vi "FilterRowData.vi"(4 "Row Filter":T1, 5 "error in (no error)":errorcluster, 7 "Ignore?":bool, 8 "Row XML Node":refnum<k20>) -> (0 "error out":errorcluster, 1 "Number Out":i32, 2 "Row Data":string[](array[string]), 3 "XML Node Out":refnum<k20>)   [LabVIEW 2013]
uses:
  RowDataFilter.ctl
  XML.lvlib
  <resource>/objmgr/DOMUserDefRef.rc
panel:
  # "Input"
  # "Output"
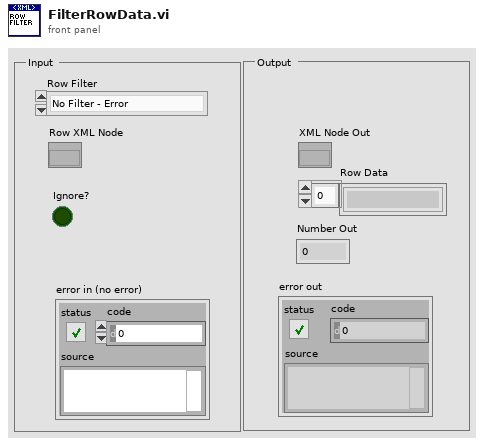
[diagram p1: front panel]
types:
  T1 = typedef "RowDataFilter.ctl" = enum16{"No Filter - Error", "Row Values", "Row Data", "#Rows Repeated", "#Columns Repeated"}
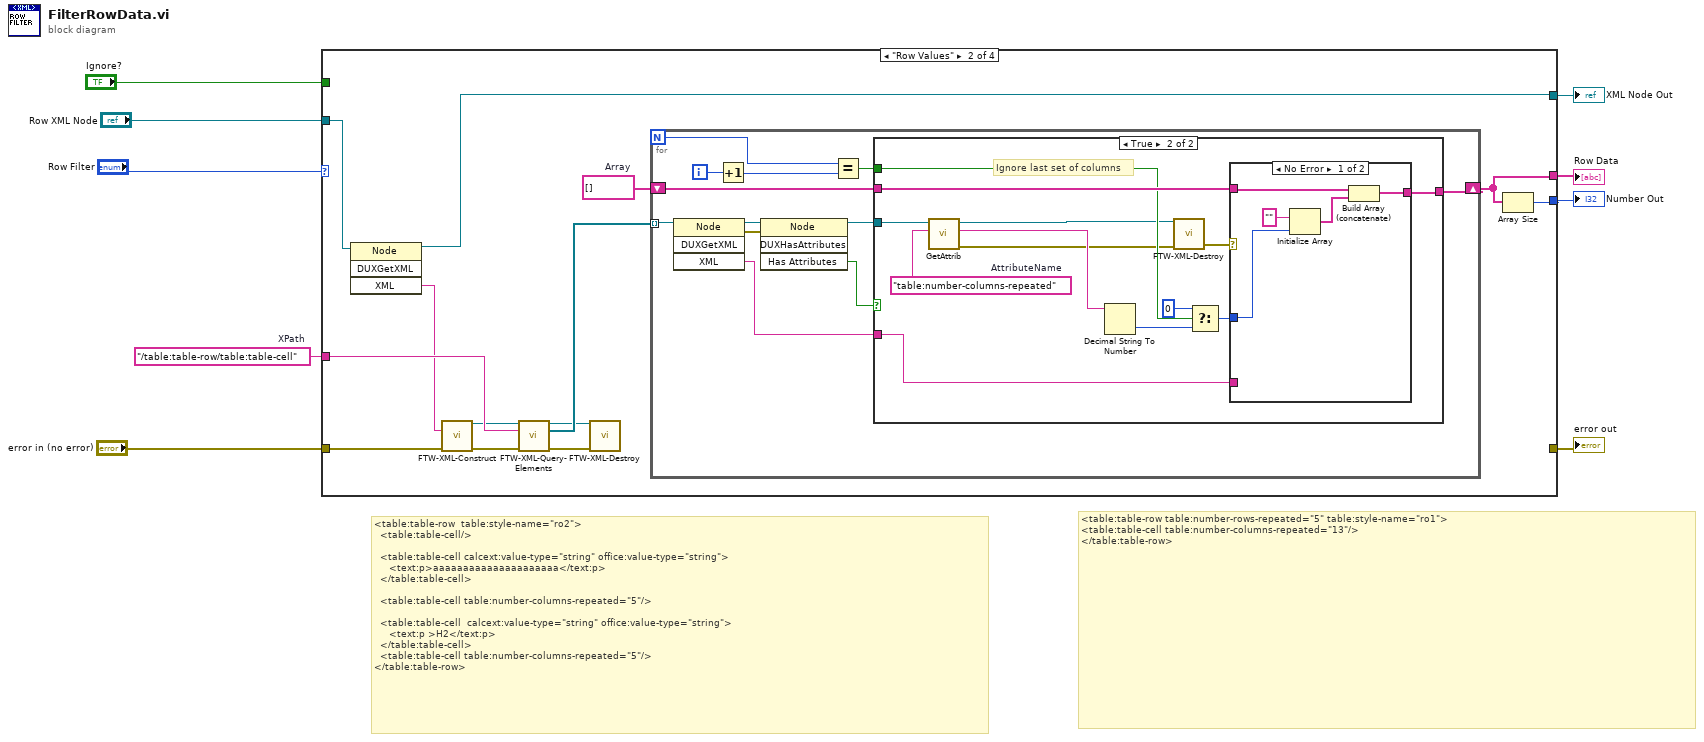
[diagram p0: block diagram]
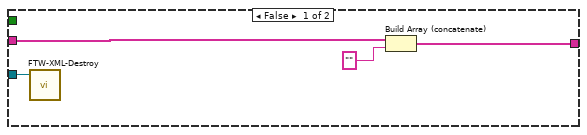
[diagram p3: hidden frame]
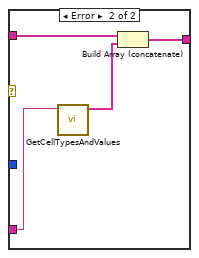
[diagram p4: hidden frame]
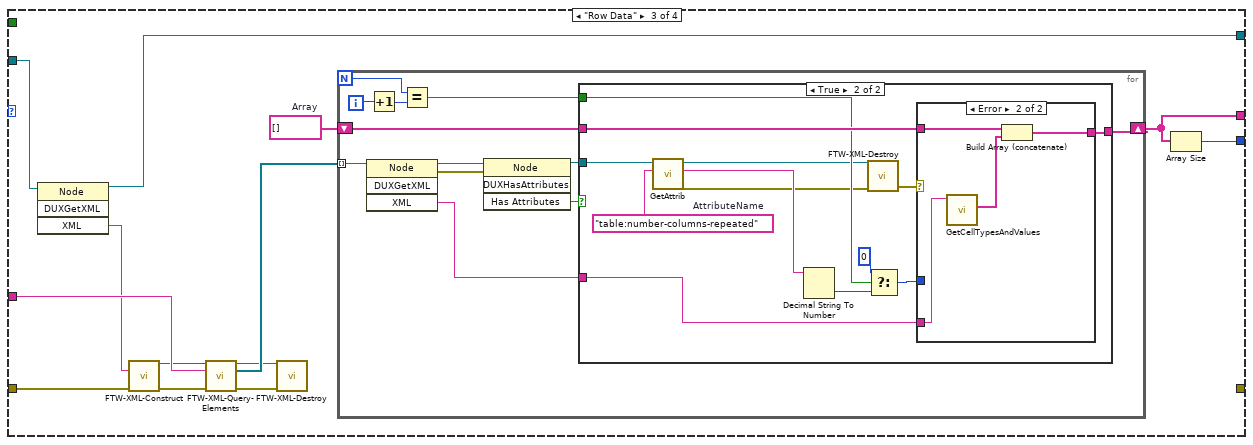
[diagram p5: hidden frame]
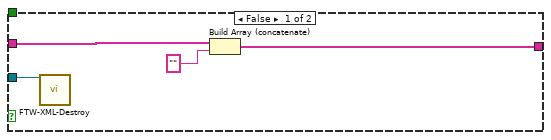
[diagram p6: hidden frame]
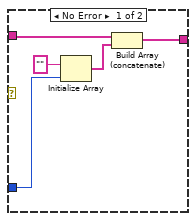
[diagram p7: hidden frame]
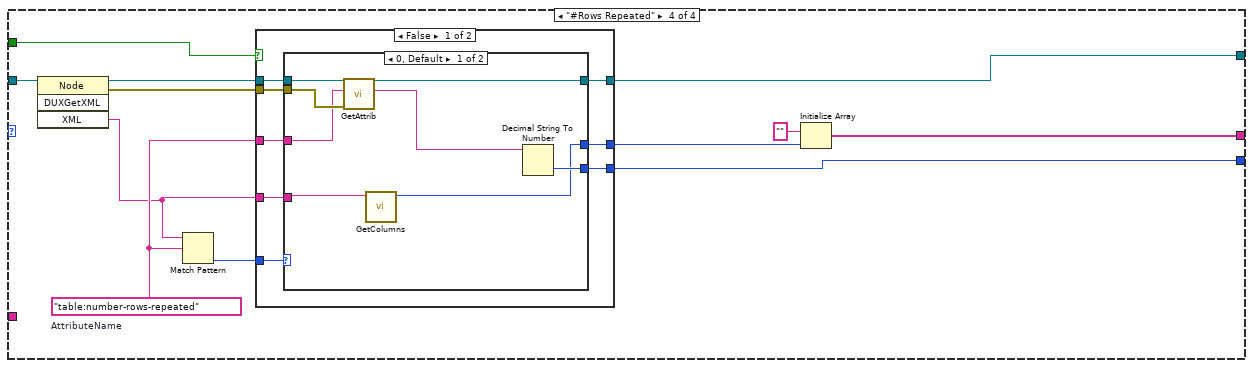
[diagram p8: hidden frame]
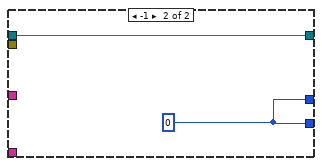
[diagram p9: hidden frame]
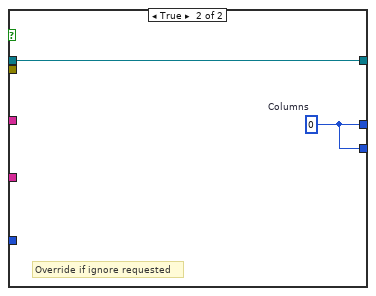
[diagram p10: hidden frame]
diagram:
  w1 = "/table:table-row/table:table-cell"  # XPath
  # "<table:table-row table:number-rows-repeated=\"5\" table:style-name=\"ro1\">\n<table:table-cell table:number-columns-repeated=\"13\"/>\n</table:table-row>"
  # "<table:table-row  table:style-name=\"ro2\">\n  <table:table-cell/>\n  \n  <table:table-cell calcext:value-type=\"string\" office:value-type=\"string\">           \n     <text:p>aaaaaaaaaaaaaaaaaaaaa</text:p>\n  </table:table-cell>\n  \n  <table:table-cell table:number-columns-repeated=\"5\"/>\n  \n  <table:table-cell  calcext:value-type=\"string\" office:value-type=\"string\">\n     <text:p >H2</text:p>\n  </table:table-cell>\n  <table:table-cell table:number-columns-repeated=\"5\"/>\n</table:table-row>"
  n1 = case shown="\"Row Values\"" "Row Filter" {
    tunnel: "error in (no error)" -> [w10 w17 w68 _]
    tunnel: "Row XML Node" -> [w11 w16 w67 w125]
    tunnel: [w11 w14 w65 w120] -> w6
    tunnel: [w10 _ _ _] -> w5
    tunnel: w1 -> [_ w24 w75 _]
    tunnel: [_ w21 w72 w122] -> w4
    tunnel: [_ w20 w71 w121] -> w3
    tunnel: "Ignore?" -> [_ _ _ w114]
    frame "No Filter - Error", Default {
    }
    frame "Row Values" {
      w22 = string[] []  # Array
      n2 = invoke class="Node" method="DUXGetXML"(reference=w16) -> (reference out=w14:refnum<k20>, "XML"=w15:string)  [unwired: 3 in, 2 out]
      n3 = call "FTW-XML-Construct.vi"("XML String"=w15, "error in"=w17) -> ("XML Document"=w19:refnum<k20>, "error out"=w18:errorcluster)  [unwired: 12 in]
      n4 = call "FTW-XML-Query-Elements.vi"("XML Node"=w19, "XPath Query"=w24, "error in"=w18) -> ("XML Node out"=w13:refnum<k20>, "Matching Nodes"=w23:refnum<k20>[], "error out"=w12:errorcluster)  [unwired: 9 in, 1 out]
      n5 = call "FTW-XML-Destroy.vi"("XML Node"=w13, "error in"=w12) -> ()  [unwired: 13 in, 1 out]
      n6 = for {
        N -> [w29]
        tunnel: w23 -> [w27] mode=indexing
        shift-right: [w33] -> w21
        shift-left: w22 -> [w34]
        i -> [w31]
        n7 = invoke class="Node" method="DUXGetXML"(reference=w27) -> (reference out=w26:refnum<k20>, error out=w25:errorcluster, "XML"=w32:string)  [unwired: 3 in, 1 out]
        n8 = Increment(x=w31) -> (x+1=w30:i32)
        n9 = invoke class="Node" method="DUXHasAttributes"(reference=w26, error in=w25) -> (reference out=w35:refnum<k20>, "Has Attributes"=w36:bool)  [unwired: 2 in, 2 out]
        n10 = Equal?(x=w29, y=w30) -> (x = y?=w28:bool)
        n11 = case shown="True" w36 {
          tunnel: w35 -> [w37 w50]
          tunnel: w34 -> [w40 w53]
          tunnel: [w38 w52] -> w33
          tunnel: w32 -> [_ w51]
          tunnel: w28 -> [_ w46]
          frame False {
            n12 = call "FTW-XML-Destroy.vi"("XML Node"=w37) -> ()  [unwired: 14 in, 1 out]
            n13 = Build Array (concatenate)(w40, "") -> (w38:string[])
          }
          frame True {
            w48 = "table:number-columns-repeated"  # AttributeName
            # "Ignore last set of columns"
            n14 = call "GetAttrib.vi"("Attrib"=w48, "Refnum in"=w50) -> ("error out"=w42:errorcluster, "Value"=w49:string, "Refnum out"=w41:refnum<k20>)  [unwired: 7 in]
            n15 = Decimal String To Number(string=w49) -> (number=w47:i32)  [unwired: 2 in, 1 out]
            n16 = call "FTW-XML-Destroy.vi"("XML Node"=w41, "error in"=w42) -> ("error out"=w43:errorcluster)  [unwired: 13 in]
            n17 = Select(t=0, s=w46, f=w47) -> (s? t:f=w44:i32)
            n18 = case shown="No Error" w43 {
              tunnel: w53 -> [w58 w61]
              tunnel: [w57 w60] -> w52
              tunnel: w44 -> [w55 _]
              tunnel: w51 -> [_ w59]
              frame No Error {
                n19 = Initialize Array("" ("Data Out"), w55) -> (w54:string[])
                n20 = Build Array (concatenate)(w58, w54) -> (w57:string[])
              }
              frame Error {
                n21 = call "GetCellTypesAndValues.vi"("XML"=w59) -> ("Value"=w62:string[])  [unwired: 9 in, 1 out]
                n22 = Build Array (concatenate)(w61, w62) -> (w60:string[])
              }
            }
          }
        }
      }
      n23 = Array Size(array=w21) -> (size(s)=w20:i32)
    }
    frame "Row Data" {
      w73 = string[] []  # Array
      n24 = invoke class="Node" method="DUXGetXML"(reference=w67) -> (reference out=w65:refnum<k20>, "XML"=w66:string)  [unwired: 3 in, 2 out]
      n25 = call "FTW-XML-Construct.vi"("XML String"=w66, "error in"=w68) -> ("XML Document"=w70:refnum<k20>, "error out"=w69:errorcluster)  [unwired: 12 in]
      n26 = call "FTW-XML-Query-Elements.vi"("XML Node"=w70, "XPath Query"=w75, "error in"=w69) -> ("XML Node out"=w64:refnum<k20>, "Matching Nodes"=w74:refnum<k20>[], "error out"=w63:errorcluster)  [unwired: 9 in, 1 out]
      n27 = call "FTW-XML-Destroy.vi"("XML Node"=w64, "error in"=w63) -> ()  [unwired: 13 in, 1 out]
      n28 = for {
        N -> [w80]
        tunnel: w74 -> [w83] mode=indexing
        shift-right: [w84] -> w72
        shift-left: w73 -> [w85]
        i -> [w79]
        n29 = invoke class="Node" method="DUXGetXML"(reference=w83) -> (reference out=w77:refnum<k20>, error out=w76:errorcluster, "XML"=w82:string)  [unwired: 3 in, 1 out]
        n30 = Increment(x=w79) -> (x+1=w81:i32)
        n31 = Equal?(x=w80, y=w81) -> (x = y?=w78:bool)
        n32 = invoke class="Node" method="DUXHasAttributes"(reference=w77, error in=w76) -> (reference out=w86:refnum<k20>, "Has Attributes"=w87:bool)  [unwired: 2 in, 2 out]
        n33 = case shown="True" w87 {
          tunnel: w86 -> [w88 w104]
          tunnel: w85 -> [w91 w103]
          tunnel: [w89 w102] -> w84
          tunnel: w82 -> [_ w100]
          tunnel: w78 -> [_ w97]
          frame False {
            n34 = call "FTW-XML-Destroy.vi"("XML Node"=w88) -> ()  [unwired: 14 in, 1 out]
            n35 = Build Array (concatenate)(w91, "") -> (w89:string[])
          }
          frame True {
            w99 = "table:number-columns-repeated"  # AttributeName
            n36 = call "GetAttrib.vi"("Attrib"=w99, "Refnum in"=w104) -> ("error out"=w93:errorcluster, "Value"=w101:string, "Refnum out"=w92:refnum<k20>)  [unwired: 7 in]
            n37 = Decimal String To Number(string=w101) -> (number=w98:i32)  [unwired: 2 in, 1 out]
            n38 = call "FTW-XML-Destroy.vi"("XML Node"=w92, "error in"=w93) -> ("error out"=w94:errorcluster)  [unwired: 13 in]
            n39 = Select(t=0, s=w97, f=w98) -> (s? t:f=w95:i32)
            n40 = case shown="Error" w94 {
              tunnel: w103 -> [w109 w113]
              tunnel: [w108 w112] -> w102
              tunnel: w95 -> [w106 _]
              tunnel: w100 -> [_ w111]
              frame No Error {
                n41 = Initialize Array("" ("Data Out"), w106) -> (w105:string[])
                n42 = Build Array (concatenate)(w109, w105) -> (w108:string[])
              }
              frame Error {
                n43 = call "GetCellTypesAndValues.vi"("XML"=w111) -> ("Type"=w110:string[])  [unwired: 9 in, 1 out]
                n44 = Build Array (concatenate)(w113, w110) -> (w112:string[])
              }
            }
          }
        }
      }
      n45 = Array Size(array=w72) -> (size(s)=w71:i32)
    }
    frame "#Rows Repeated" {
      w117 = "table:number-rows-repeated"  # AttributeName
      n46 = invoke class="Node" method="DUXGetXML"(reference=w125) -> (reference out=w119:refnum<k20>, error out=w124:errorcluster, "XML"=w116:string)  [unwired: 3 in, 1 out]
      n47 = Match Pattern(string=w116, regular expression=w117) -> (offset past match=w118:i32)  [unwired: 1 in, 3 out]
      n48 = case shown="False" w114 {
        tunnel: w124 -> [w133 _]
        tunnel: [w132 w144] -> w121
        tunnel: [w131 w145] -> w120
        tunnel: w119 -> [w130 w145]
        tunnel: w118 -> [w129 _]
        tunnel: w117 -> [w128 _]
        tunnel: w116 -> [w127 _]
        tunnel: [w126 w144] -> w115
        frame False {
          n49 = case shown="0, Default" w129 {
            tunnel: w133 -> [w136 _]
            tunnel: [w141 w142] -> w132
            tunnel: [w137 w143] -> w131
            tunnel: w130 -> [w138 w143]
            tunnel: w128 -> [w135 _]
            tunnel: w127 -> [w140 _]
            tunnel: [w139 w142] -> w126
            frame 0, Default {
              n50 = call "GetAttrib.vi"("error in (no error)"=w136, "Attrib"=w135, "Refnum in"=w138) -> ("Value"=w134:string, "Refnum out"=w137:refnum<k20>)  [unwired: 6 in, 1 out]
              n51 = call "GetColumns.vi"("XML"=w140) -> ("#Columns"=w139:i32)  [unwired: 9 in, 1 out]
              n52 = Decimal String To Number(string=w134) -> (number=w141:i32)  [unwired: 2 in, 1 out]
            }
            frame -1 {
              w142 = 0
            }
          }
        }
        frame True {
          w144 = 0  # Columns
          # "Override if ignore requested"
        }
      }
      n53 = Initialize Array("" ("Data Out"), w115) -> (w122:string[])
    }
  }
  "error out" <- w5
  "Number Out" <- w3
  "XML Node Out" <- w6
  "Row Data" <- w4
